vi "Lab Panel V4.90.vi"() -> ()   [LabVIEW 2013] (continued)
              n212 = Bundle(cluster=w241, "Tmp Live"=w237, "Tmp Neut"=w236) -> (w239:T2)  [unwired: 3 in]
              n213 = local write "TEMP LA02"(w243) -> ()
              n214 = local write "SIG LAB02-1"(w239) -> ()
              n215 = local write "SIG LAB02-2"(w238) -> ()
            }
            frame #4 {
              w254 = 0
              n216 = local read "LAB03 TEMP"() -> (w256:T12)
              n217 = Unbundle By Name(w256) -> ("T1 Live"=w249:dbl, "T1 Neut"=w248:dbl, "T2 Live"=w247:dbl, "T2 Neut"=w246:dbl)  [unwired: 2 out]
              n218 = local read "SIG LAB03-1"() -> (w253:T2)
              n219 = local read "SIG LAB03-2"() -> (w252:T2)
              n220 = local read "TEMP LA03"() -> (w257:T9)
              n221 = Bundle By Name(cluster=w257, "TL-1"=w249, "TN-1"=w248, "TL-2"=w247, "TN-2"=w246, "TL -1COUNT"=w254, "TN-1 COUNT"=w254, "TL-2 COUNT"=w254, "TN-2 COUNT"=w254) -> (w255:T9)
              n222 = Bundle(cluster=w252, "Tmp Live"=w247, "Tmp Neut"=w246) -> (w250:T2)  [unwired: 3 in]
              n223 = Bundle(cluster=w253, "Tmp Live"=w249, "Tmp Neut"=w248) -> (w251:T2)  [unwired: 3 in]
              n224 = local write "TEMP LA03"(w255) -> ()
              n225 = local write "SIG LAB03-2"(w250) -> ()
              n226 = local write "SIG LAB03-1"(w251) -> ()
            }
            frame #5 {
              w266 = 0
              n227 = local read "LAB04 TEMP"() -> (w268:T12)
              n228 = Unbundle By Name(w268) -> ("T1 Live"=w261:dbl, "T1 Neut"=w260:dbl, "T2 Live"=w259:dbl, "T2 Neut"=w258:dbl)  [unwired: 2 out]
              n229 = local read "SIG LAB04-2"() -> (w264:T2)
              n230 = local read "SIG LAB04-1"() -> (w265:T2)
              n231 = local read "TEMP LA04"() -> (w269:T9)
              n232 = Bundle By Name(cluster=w269, "TL-1"=w261, "TN-1"=w260, "TL-2"=w259, "TN-2"=w258, "TL -1COUNT"=w266, "TN-1 COUNT"=w266, "TL-2 COUNT"=w266, "TN-2 COUNT"=w266) -> (w267:T9)
              n233 = Bundle(cluster=w264, "Tmp Live"=w259, "Tmp Neut"=w258) -> (w262:T2)  [unwired: 3 in]
              n234 = Bundle(cluster=w265, "Tmp Live"=w261, "Tmp Neut"=w260) -> (w263:T2)  [unwired: 3 in]
              n235 = local write "SIG LAB04-2"(w262) -> ()
              n236 = local write "TEMP LA04"(w267) -> ()
              n237 = local write "SIG LAB04-1"(w263) -> ()
            }
            frame #6 {
              w278 = 0
              n238 = local read "LAB05 TEMP"() -> (w280:T12)
              n239 = Unbundle By Name(w280) -> ("T1 Live"=w273:dbl, "T1 Neut"=w272:dbl, "T2 Live"=w271:dbl, "T2 Neut"=w270:dbl)  [unwired: 2 out]
              n240 = local read "SIG LAB05-2"() -> (w276:T2)
              n241 = local read "SIG LAB05-1"() -> (w277:T2)
              n242 = local read "TEMP LA05"() -> (w281:T9)
              n243 = Bundle By Name(cluster=w281, "TL-1"=w273, "TN-1"=w272, "TL-2"=w271, "TN-2"=w270, "TL -1COUNT"=w278, "TN-1 COUNT"=w278, "TL-2 COUNT"=w278, "TN-2 COUNT"=w278) -> (w279:T9)
              n244 = Bundle(cluster=w276, "Tmp Live"=w271, "Tmp Neut"=w270) -> (w274:T2)  [unwired: 3 in]
              n245 = Bundle(cluster=w277, "Tmp Live"=w273, "Tmp Neut"=w272) -> (w275:T2)  [unwired: 3 in]
              n246 = local write "SIG LAB05-2"(w274) -> ()
              n247 = local write "SIG LAB05-1"(w275) -> ()
              n248 = local write "TEMP LA05"(w279) -> ()
            }
          }
        }
        frame #8 {
          # "enable front panel, all settings done"
          n249 = property on="Tab Control 2" class="TabCtl (strict)"("DisabledEnum"=T16."Enabled" ("Disabled")) -> ()  [unwired: 2 in, 2 out]
          n250 = property on="Tab Control 2" class="TabCtl (strict)"("Value"=0) -> ()  [unwired: 2 in, 2 out]
        }
        frame #9 {
          n251 = property on="Tab Control 2" class="TabCtl (strict)"("Value"=0) -> ()  [unwired: 2 in, 2 out]
        }
      }
    }
    frame #2 {
      n252 = node-c288("loop  delay(mS)") -> (w287:T17)  [unwired: 3 in]
      n253 = timed-loop {
        timing: w287 -> [_]
        timing-out: [_] -> w286
        i -> [w309]
        stop <- "stop" stop-if-true
        n254 = node-c288() -> ()  [unwired: 1 in, 1 out]
        n255 = global write "Global display 1.vi" "stop disp"("stop") -> ()
        n256 = local read "SELECT LAB05-2"() -> (w289:T3)
        n257 = local read "SELECT LAB05-1"() -> (w290:T3)
        n258 = local read "SELECT LAB04-2"() -> (w291:T3)
        n259 = local read "SELECT LAB03-1"() -> (w294:T3)
        n260 = local read "SELECT LAB02-2"() -> (w295:T3)
        n261 = local read "SELECT LAB01-1"() -> (w298:T3)
        n262 = local read "SELECT LAB03-2"() -> (w293:T3)
        n263 = local read "SELECT LAB01-2"() -> (w297:T3)
        n264 = local read "SELECT LAB04-1"() -> (w292:T3)
        n265 = local read "SELECT LAB02-1"() -> (w296:T3)
        n266 = local read "run lab03-2"() -> (w303:bool)
        n267 = local read "run lab04-1"() -> (w302:bool)
        n268 = local read "run lab05-1"() -> (w300:bool)
        n269 = local read "run lab04-2"() -> (w301:bool)
        n270 = local read "run lab05-2"() -> (w299:bool)
        n271 = local read "run lab03-1"() -> (w304:bool)
        n272 = local read "run lab02-2"() -> (w305:bool)
        n273 = local read "run lab02-1"() -> (w306:bool)
        n274 = local read "run lab01-1"() -> (w308:bool)
        n275 = local read "run lab01-2"() -> (w307:bool)
        n276 = stacked-sequence {
          seq-local: [_ w374 _ _ _ _ _ _ _ _ _ _ _ _ _ _ _ _ _ _ _ _ _] -> [_ _ _ _ _ w2475 _ _ _ _ _ _ _ _ _ _ _ _ _ _ _ _ _]
          seq-local: [_ w373 _ _ _ _ _ _ _ _ _ _ _ _ _ _ _ _ _ _ _ _ _] -> [_ _ _ _ _ w2474 _ _ _ _ _ _ _ _ _ _ _ _ _ _ _ _ _]
          seq-local: [_ w360 _ _ _ _ _ _ _ _ _ _ _ _ _ _ _ _ _ _ _ _ _] -> [_ _ _ _ _ w2473 _ _ _ _ _ _ _ _ _ _ _ _ _ _ _ _ _]
          seq-local: [_ w359 _ _ _ _ _ _ _ _ _ _ _ _ _ _ _ _ _ _ _ _ _] -> [_ _ _ _ _ w2472 _ _ _ _ _ _ _ _ _ _ _ _ _ _ _ _ _]
          seq-local: [_ w358 _ _ _ _ _ _ _ _ _ _ _ _ _ _ _ _ _ _ _ _ _] -> [_ _ _ _ _ w2471 _ _ _ _ _ _ _ _ _ _ _ _ _ _ _ _ _]
          seq-local: [_ w357 _ _ _ _ _ _ _ _ _ _ _ _ _ _ _ _ _ _ _ _ _] -> [_ _ _ _ _ w2470 _ _ _ _ _ _ _ _ _ _ _ _ _ _ _ _ _]
          seq-local: [_ w356 _ _ _ _ _ _ _ _ _ _ _ _ _ _ _ _ _ _ _ _ _] -> [_ _ _ _ _ w2469 _ _ _ _ _ _ _ _ _ _ _ _ _ _ _ _ _]
          seq-local: [_ w355 _ _ _ _ _ _ _ _ _ _ _ _ _ _ _ _ _ _ _ _ _] -> [_ _ _ _ _ w2468 _ _ _ _ _ _ _ _ _ _ _ _ _ _ _ _ _]
          seq-local: [_ w354 _ _ _ _ _ _ _ _ _ _ _ _ _ _ _ _ _ _ _ _ _] -> [_ _ _ _ _ w2467 _ _ _ _ _ _ _ _ _ _ _ _ _ _ _ _ _]
          seq-local: [_ w353 _ _ _ _ _ _ _ _ _ _ _ _ _ _ _ _ _ _ _ _ _] -> [_ _ _ _ _ w2466 _ _ _ _ _ _ _ _ _ _ _ _ _ _ _ _ _]
          tunnel: w308 -> [_ _ w390 w638 w2065 w2495 w2810 w3297 _ _ _ _ w3722 _ w4679 _ _ w4966 w5269 w5451 _ _ _]
          tunnel: w307 -> [_ _ w389 w636 w2064 w2494 w2811 w3296 _ _ _ _ w3721 _ w4677 _ _ w4965 w5268 w5449 _ _ _]
          tunnel: w306 -> [_ _ w388 w634 w2063 w2493 w2809 w3295 _ _ _ _ w3720 _ w4675 _ _ w4964 w5267 w5448 _ _ _]
          tunnel: w305 -> [_ _ w387 w632 w2062 w2492 w2808 w3294 _ _ _ _ w3719 _ w4673 _ _ w4963 w5266 w5447 _ _ _]
          tunnel: w304 -> [_ _ w386 w630 w2061 w2491 w2807 w3293 _ _ _ _ w3718 _ w4671 _ _ w4962 w5265 w5446 _ _ _]
          tunnel: w303 -> [_ _ w385 w628 w2060 w2490 w2806 w3292 _ _ _ _ w3717 _ w4669 _ _ w4961 w5264 w5445 _ _ _]
          tunnel: w302 -> [_ _ w384 w626 w2059 w2489 w2805 w3291 _ _ _ _ w3716 _ w4667 _ _ w4960 w5263 w5444 _ _ _]
          tunnel: w301 -> [_ _ w383 w624 w2058 w2488 w2804 w3290 _ _ _ _ w3715 _ w4665 _ _ w4959 w5262 w5443 _ _ _]
          tunnel: w300 -> [_ _ w382 w622 w2057 w2487 w2803 w3289 _ _ _ _ w3714 _ w4663 _ _ w4958 w5261 w5442 _ _ _]
          tunnel: w299 -> [_ _ w381 w620 w2056 w2486 w2802 w3288 _ _ _ _ w3713 _ w4661 _ _ w4957 w5260 w5441 _ _ _]
          tunnel: w298 -> [_ _ _ w637 w2055 w2485 _ _ _ _ _ _ _ _ w4681 _ _ _ _ _ w5789 _ _]
          tunnel: w297 -> [_ _ _ w635 w2054 w2484 _ _ _ _ _ _ _ _ w4676 _ _ _ _ _ w5788 _ _]
          tunnel: w296 -> [_ _ _ w633 w2053 w2483 _ _ _ _ _ _ _ _ w4674 _ _ _ _ _ w5787 _ _]
          tunnel: w295 -> [_ _ _ w631 w2052 w2482 _ _ _ _ _ _ _ _ w4672 _ _ _ _ _ w5786 _ _]
          tunnel: w294 -> [_ _ _ w629 w2051 w2481 _ _ _ _ _ _ _ _ w4670 _ _ _ _ _ w5785 _ _]
          tunnel: w293 -> [_ _ _ w627 w2050 w2480 _ _ _ _ _ _ _ _ w4668 _ _ _ _ _ w5784 _ _]
          tunnel: w292 -> [_ _ _ w625 w2049 w2479 _ _ _ _ _ _ _ _ w4666 _ _ _ _ _ w5783 _ _]
          tunnel: w291 -> [_ _ _ w623 w2048 w2478 _ _ _ _ _ _ _ _ w4664 _ _ _ _ _ w5782 _ _]
          tunnel: w290 -> [_ _ _ w621 w2047 w2477 _ _ _ _ _ _ _ _ w4662 _ _ _ _ _ w5781 _ _]
          tunnel: w289 -> [_ _ _ w619 w2046 w2476 _ _ _ _ _ _ _ _ w4660 _ _ _ _ _ w5780 _ _]
          frame #0 {
            w316 = FALSE
            w321 = 0.5
            # "set up cycle control"
            n277 = local read "jig cycle"() -> (w320:dbl)
            n278 = local read "Amps Fail level"() -> (w314:dbl)
            n279 = Divide(x="JIG ON TIME (S)", y=w321) -> (x/y=→"on loops":dbl)
            n280 = Divide(x="JIG OFF TIME (S)", y=w321) -> (x/y=→"off loops":dbl)
            n281 = global write "Global display 3.vi" "Amps Fail"(w314) -> ()
            n282 = Increment(x=w320) -> (x+1=w319:dbl)
            n283 = local write "TEMP"(w316) -> ()
            n284 = local write "AI"(w316) -> ()
            n285 = local read "Network Directory"() -> (w313:path)
            n286 = local write "jig cycle"(w319) -> ()
            n287 = call "sub vi - check network dir v2.vi"("PATH"=w313) -> ("error"=w312:bool)  [unwired: 10 in]
            n288 = local write "network error"(w312) -> ()
            n289 = global write "Global display 3.vi" "network drive"(w312) -> ()
            n290 = event shown="[1] \"ADMIN\": Value Change" {
              selector: _ -> [_ _]
              dyn-events: _ -> [_ _]
              timeout: 10 -> [_ _]
              event Timeout {
                n291 = event-data() -> ()  [unwired: 1 in, 3 out]
              }
              event "ADMIN": Value Change {
                n292 = event-data() -> ()  [unwired: 1 in, 6 out]
                n293 = stacked-sequence {
                  seq-local: [_ w325 _] -> [_ _ w326]
                  frame #0 {
                    n294 = global write "Global 1.vi" "password"("9949") -> ()
                  }
                  frame #1 {
                    n295 = call "sub vi - password 1.vi"() -> ("RESULT"=w325:bool)  [unwired: 11 in]
                  }
                  frame #2 {
                    w328 = FALSE
                    n296 = property on="Tab Control 2" class="TabCtl (strict)"() -> ("Pages"=w332:refnum<vi>[])  [unwired: 2 in, 2 out]
                    n297 = Select(t=TRUE, s=w326, f=w328) -> (s? t:f=w327:bool)
                    n298 = Index Array(array=w332, index=8) -> (element=w330:refnum<vi>)
                    n299 = property class="Page"(reference=w330, "PageVis"=w327) -> ()  [unwired: 1 in, 2 out]
                    n300 = local write "ADMIN"(w328) -> ()
                  }
                }
              }
            }
          }
          frame #1 {
            w370 = 60.0
            # "convert temperature rise minutes to cycles"
            n301 = local read "SET LAB05-2"() -> (w334:T5)
            n302 = local read "SET LAB05-1"() -> (w336:T5)
            n303 = local read "SET LAB04-2"() -> (w338:T5)
            n304 = local read "SET LAB01-1"() -> (w352:T5)
            n305 = local read "SET LAB01-2"() -> (w350:T5)
            n306 = local read "SET LAB02-2"() -> (w346:T5)
            n307 = local read "SET LAB04-1"() -> (w340:T5)
            n308 = local read "SET LAB03-1"() -> (w344:T5)
            n309 = local read "SET LAB03-2"() -> (w342:T5)
            n310 = local read "SET LAB02-1"() -> (w348:T5)
            n311 = local read "JIG OFF TIME (S)"() -> (w375:dbl)
            n312 = local read "JIG ON TIME (S)"() -> (w376:dbl)
            n313 = Unbundle(w334) -> ("T-RISE mins"=w333:dbl)  [unwired: 4 out]
            n314 = Unbundle(w336) -> ("T-RISE mins"=w335:dbl)  [unwired: 4 out]
            n315 = Unbundle(w352) -> ("T-RISE mins"=w351:dbl)  [unwired: 4 out]
            n316 = Unbundle(w338) -> ("T-RISE mins"=w337:dbl)  [unwired: 4 out]
            n317 = Unbundle(w350) -> ("T-RISE mins"=w349:dbl)  [unwired: 4 out]
            n318 = Unbundle(w348) -> ("T-RISE mins"=w347:dbl)  [unwired: 4 out]
            n319 = Unbundle(w340) -> ("T-RISE mins"=w339:dbl)  [unwired: 4 out]
            n320 = Unbundle(w346) -> ("T-RISE mins"=w345:dbl)  [unwired: 4 out]
            n321 = Unbundle(w342) -> ("T-RISE mins"=w341:dbl)  [unwired: 4 out]
            n322 = Unbundle(w344) -> ("T-RISE mins"=w343:dbl)  [unwired: 4 out]
            n323 = Add(x=w376, y=w375) -> (x+y=w369:dbl)
            n324 = Multiply(x=w370, y=w341) -> (x*y=w365:dbl)
            n325 = Multiply(x=w370, y=w339) -> (x*y=w364:dbl)
            n326 = Multiply(x=w370, y=w337) -> (x*y=w363:dbl)
            n327 = Multiply(x=w370, y=w335) -> (x*y=w362:dbl)
            n328 = Multiply(x=w370, y=w333) -> (x*y=w361:dbl)
            n329 = Multiply(x=w370, y=w349) -> (x*y=w371:dbl)
            n330 = Multiply(x=w370, y=w343) -> (x*y=w366:dbl)
            n331 = Multiply(x=w370, y=w351) -> (x*y=w372:dbl)
            n332 = Multiply(x=w370, y=w347) -> (x*y=w368:dbl)
            n333 = Multiply(x=w370, y=w345) -> (x*y=w367:dbl)
            n334 = Divide(x=w362, y=w369) -> (x/y=w354:dbl)
            n335 = Divide(x=w363, y=w369) -> (x/y=w355:dbl)
            n336 = Divide(x=w364, y=w369) -> (x/y=w356:dbl)
            n337 = Divide(x=w361, y=w369) -> (x/y=w353:dbl)
            n338 = Divide(x=w366, y=w369) -> (x/y=w358:dbl)
            n339 = Divide(x=w372, y=w369) -> (x/y=w374:dbl)
            n340 = Divide(x=w371, y=w369) -> (x/y=w373:dbl)
            n341 = Divide(x=w368, y=w369) -> (x/y=w360:dbl)
            n342 = Divide(x=w367, y=w369) -> (x/y=w359:dbl)
            n343 = Divide(x=w365, y=w369) -> (x/y=w357:dbl)
          }
          frame #2 {
            # "control cycle loops"
            n344 = local read "JIG OFF TIME (S)"() -> (w379:dbl)
            n345 = local read "JIG ON TIME (S)"() -> (w378:dbl)
            n346 = local read "jig cycle"() -> (w392:dbl)
            n347 = local read "on loops"() -> (w394:dbl)
            n348 = local read "off loops"() -> (w393:dbl)
            n349 = Add(x=w379, y=w378) -> (x+y=w377:dbl)
            n350 = Add(x=w394, y=w393) -> (x+y=w380:dbl)
            n351 = Greater Or Equal?(x=w392, y=w380) -> (x >= y?=w391:bool)
            n352 = case shown="True" w391 {
              tunnel: w390 -> [_ w428]
              tunnel: w389 -> [_ w427]
              tunnel: w388 -> [_ w426]
              tunnel: w387 -> [_ w425]
              tunnel: w386 -> [_ w424]
              tunnel: w385 -> [_ w423]
              tunnel: w384 -> [_ w422]
              tunnel: w383 -> [_ w421]
              tunnel: w382 -> [_ w420]
              tunnel: w381 -> [_ w419]
              tunnel: w377 -> [_ w418]
              frame False {
              }
              frame True {
                # "increment cycle value and convert cycles to minutes for temp rise"
                n353 = stacked-sequence {
                  frame #0 {
                    n354 = local read "Panel #"() -> (w431:dbl)
                    n355 = Increment(x=w431) -> (x+1=w430:dbl)
                    n356 = local write "Panel #"(w430) -> ()
                  }
                  frame #1 {
                    n357 = local read "Panel #"() -> (w432:dbl)
                    n358 = Greater?(x=w432, y=5) -> (0:w434:bool)
                    n359 = case shown="True" w434 {
                      frame False {
                      }
                      frame True {
                        n360 = local write "Panel #"(1) -> ()
                      }
                    }
                  }
                }
                n361 = local read "JIG RELAY CYCLES"() -> (w417:T8)
                n362 = local read "Panel #"() -> (→"Tmp Upd":dbl)
                n363 = Unbundle By Name(w417) -> ("LAB01-1"=w415:dbl, "LAB01-2"=w413:dbl, "LAB02-1"=w411:dbl, "LAB02-2"=w409:dbl, "LAB03-1"=w407:dbl, "LAB03-2"=w405:dbl, "LAB04-1"=w403:dbl, "LAB04-2"=w401:dbl, "LAB05-1"=w399:dbl, "LAB05-2"=w397:dbl)
                n364 = stacked-sequence {
                  tunnel: w428 -> [w446 _ _ _ _ _ _ _ _ _]
                  tunnel: w427 -> [_ w463 _ _ _ _ _ _ _ _]
                  tunnel: w426 -> [_ _ w480 _ _ _ _ _ _ _]
                  tunnel: w425 -> [_ _ _ w497 _ _ _ _ _ _]
                  tunnel: w424 -> [_ _ _ _ w514 _ _ _ _ _]
                  tunnel: w423 -> [_ _ _ _ _ w531 _ _ _ _]
                  tunnel: w422 -> [_ _ _ _ _ _ w548 _ _ _]
                  tunnel: w421 -> [_ _ _ _ _ _ _ w565 _ _]
                  tunnel: w420 -> [_ _ _ _ _ _ _ _ w582 _]
                  tunnel: w419 -> [_ _ _ _ _ _ _ _ _ w599]
                  tunnel: w418 -> [w443 w460 w477 w494 w511 w528 w545 w562 w579 w596]
                  tunnel: w415 -> [w437 _ _ _ _ _ _ _ _ _]
                  tunnel: [w436 _ _ _ _ _ _ _ _ _] -> w414
                  tunnel: w413 -> [_ w454 _ _ _ _ _ _ _ _]
                  tunnel: [_ w453 _ _ _ _ _ _ _ _] -> w412
                  tunnel: w411 -> [_ _ w471 _ _ _ _ _ _ _]
                  tunnel: [_ _ w470 _ _ _ _ _ _ _] -> w410
                  tunnel: w409 -> [_ _ _ w488 _ _ _ _ _ _]
                  tunnel: [_ _ _ w487 _ _ _ _ _ _] -> w408
                  tunnel: w407 -> [_ _ _ _ w505 _ _ _ _ _]
                  tunnel: [_ _ _ _ w504 _ _ _ _ _] -> w406
                  tunnel: w405 -> [_ _ _ _ _ w522 _ _ _ _]
                  tunnel: [_ _ _ _ _ w521 _ _ _ _] -> w404
                  tunnel: w403 -> [_ _ _ _ _ _ w539 _ _ _]
                  tunnel: [_ _ _ _ _ _ w538 _ _ _] -> w402
                  tunnel: w401 -> [_ _ _ _ _ _ _ w556 _ _]
                  tunnel: [_ _ _ _ _ _ _ w555 _ _] -> w400
                  tunnel: w399 -> [_ _ _ _ _ _ _ _ w573 _]
                  tunnel: [_ _ _ _ _ _ _ _ w572 _] -> w398
                  tunnel: w397 -> [_ _ _ _ _ _ _ _ _ w590]
                  tunnel: [_ _ _ _ _ _ _ _ _ w589] -> w396
                  frame #0 {
                    n365 = local read "DISP LAB01-1"() -> (w441:T4)
                    n366 = Unbundle(w441) -> ("CYCLE"=w442:dbl)  [unwired: 2 out]
                    n367 = case shown="True" w446 {
                      tunnel: w442 -> [w448 w452]
                      tunnel: [w448 w451] -> w440
                      tunnel: w437 -> [w447 w450]
                      tunnel: [w447 w449] -> w436
                      frame False {
                      }
                      frame True {
                        n368 = Increment(x=w450) -> (x+1=w449:dbl)
                        n369 = Increment(x=w452) -> (x+1=w451:dbl)
                      }
                    }
                    n370 = Multiply(x=w440, y=w443) -> (x*y=w444:dbl)
                    n371 = Divide(x=w444, y=60.0) -> (x/y=w439:dbl)
                    n372 = Bundle(cluster=w441, "CYCLE"=w440, "MINS"=w439) -> (w438:T4)  [unwired: 1 in]
                    n373 = local write "DISP LAB01-1"(w438) -> ()
                  }
                  frame #1 {
                    n374 = local read "DISP LAB01-2"() -> (w458:T4)
                    n375 = Unbundle(w458) -> ("CYCLE"=w459:dbl)  [unwired: 2 out]
                    n376 = case shown="True" w463 {
                      tunnel: w459 -> [w465 w469]
                      tunnel: [w465 w468] -> w456
                      tunnel: w454 -> [w464 w467]
                      tunnel: [w464 w466] -> w453
                      frame False {
                      }
                      frame True {
                        n377 = Increment(x=w467) -> (x+1=w466:dbl)
                        n378 = Increment(x=w469) -> (x+1=w468:dbl)
                      }
                    }
                    n379 = Multiply(x=w456, y=w460) -> (x*y=w461:dbl)
                    n380 = Divide(x=w461, y=60.0) -> (x/y=w455:dbl)
                    n381 = Bundle(cluster=w458, "CYCLE"=w456, "MINS"=w455) -> (w457:T4)  [unwired: 1 in]
                    n382 = local write "DISP LAB01-2"(w457) -> ()
                  }
                  frame #2 {
                    n383 = local read "DISP LAB02-1"() -> (w475:T4)
                    n384 = Unbundle(w475) -> ("CYCLE"=w476:dbl)  [unwired: 2 out]
                    n385 = case shown="True" w480 {
                      tunnel: [w482 w486] -> w473
                      tunnel: w476 -> [w482 w485]
                      tunnel: w471 -> [w481 w484]
                      tunnel: [w481 w483] -> w470
                      frame False {
                      }
                      frame True {
                        n386 = Increment(x=w484) -> (x+1=w483:dbl)
                        n387 = Increment(x=w485) -> (x+1=w486:dbl)
                      }
                    }
                    n388 = Multiply(x=w473, y=w477) -> (x*y=w478:dbl)
                    n389 = Divide(x=w478, y=60.0) -> (x/y=w472:dbl)
                    n390 = Bundle(cluster=w475, "CYCLE"=w473, "MINS"=w472) -> (w474:T4)  [unwired: 1 in]
                    n391 = local write "DISP LAB02-1"(w474) -> ()
                  }
                  frame #3 {
                    n392 = local read "DISP LAB02-2"() -> (w492:T4)
                    n393 = Unbundle(w492) -> ("CYCLE"=w493:dbl)  [unwired: 2 out]
                    n394 = case shown="True" w497 {
                      tunnel: [w499 w503] -> w491
                      tunnel: w493 -> [w499 w502]
                      tunnel: w488 -> [w498 w501]
                      tunnel: [w498 w500] -> w487
                      frame False {
                      }
                      frame True {
                        n395 = Increment(x=w501) -> (x+1=w500:dbl)
                        n396 = Increment(x=w502) -> (x+1=w503:dbl)
                      }
                    }
                    n397 = Multiply(x=w491, y=w494) -> (x*y=w495:dbl)
                    n398 = Divide(x=w495, y=60.0) -> (x/y=w490:dbl)
                    n399 = Bundle(cluster=w492, "CYCLE"=w491, "MINS"=w490) -> (w489:T4)  [unwired: 1 in]
                    n400 = local write "DISP LAB02-2"(w489) -> ()
                  }
                  frame #4 {
                    n401 = local read "DISP LAB03-1"() -> (w509:T4)
                    n402 = Unbundle(w509) -> ("CYCLE"=w510:dbl)  [unwired: 2 out]
                    n403 = case shown="True" w514 {
                      tunnel: [w516 w520] -> w506
                      tunnel: w510 -> [w516 w519]
                      tunnel: w505 -> [w515 w518]
                      tunnel: [w515 w517] -> w504
                      frame False {
                      }
                      frame True {
                        n404 = Increment(x=w518) -> (x+1=w517:dbl)
                        n405 = Increment(x=w519) -> (x+1=w520:dbl)
                      }
                    }
                    n406 = Multiply(x=w506, y=w511) -> (x*y=w512:dbl)
                    n407 = Divide(x=w512, y=60.0) -> (x/y=w507:dbl)
                    n408 = Bundle(cluster=w509, "CYCLE"=w506, "MINS"=w507) -> (w508:T4)  [unwired: 1 in]
                    n409 = local write "DISP LAB03-1"(w508) -> ()
                  }
                  frame #5 {
                    n410 = local read "DISP LAB03-2"() -> (w526:T4)
                    n411 = Unbundle(w526) -> ("CYCLE"=w527:dbl)  [unwired: 2 out]
                    n412 = case shown="True" w531 {
                      tunnel: [w533 w537] -> w525
                      tunnel: w527 -> [w533 w536]
                      tunnel: w522 -> [w532 w535]
                      tunnel: [w532 w534] -> w521
                      frame False {
                      }
                      frame True {
                        n413 = Increment(x=w535) -> (x+1=w534:dbl)
                        n414 = Increment(x=w536) -> (x+1=w537:dbl)
                      }
                    }
                    n415 = Multiply(x=w525, y=w528) -> (x*y=w529:dbl)
                    n416 = Divide(x=w529, y=60.0) -> (x/y=w524:dbl)
                    n417 = Bundle(cluster=w526, "CYCLE"=w525, "MINS"=w524) -> (w523:T4)  [unwired: 1 in]
                    n418 = local write "DISP LAB03-2"(w523) -> ()
                  }
                  frame #6 {
                    n419 = local read "DISP LAB04-1"() -> (w543:T4)
                    n420 = Unbundle(w543) -> ("CYCLE"=w544:dbl)  [unwired: 2 out]
                    n421 = case shown="True" w548 {
                      tunnel: [w550 w554] -> w541
                      tunnel: w544 -> [w550 w553]
                      tunnel: w539 -> [w549 w552]
                      tunnel: [w549 w551] -> w538
                      frame False {
                      }
                      frame True {
                        n422 = Increment(x=w552) -> (x+1=w551:dbl)
                        n423 = Increment(x=w553) -> (x+1=w554:dbl)
                      }
                    }
                    n424 = Multiply(x=w541, y=w545) -> (x*y=w546:dbl)
                    n425 = Divide(x=w546, y=60.0) -> (x/y=w540:dbl)
                    n426 = Bundle(cluster=w543, "CYCLE"=w541, "MINS"=w540) -> (w542:T4)  [unwired: 1 in]
                    n427 = local write "DISP LAB04-1"(w542) -> ()
                  }
                  frame #7 {
                    n428 = local read "DISP LAB04-2"() -> (w560:T4)
                    n429 = Unbundle(w560) -> ("CYCLE"=w561:dbl)  [unwired: 2 out]
                    n430 = case shown="True" w565 {
                      tunnel: [w567 w571] -> w558
                      tunnel: w561 -> [w567 w570]
                      tunnel: w556 -> [w566 w569]
                      tunnel: [w566 w568] -> w555
                      frame False {
                      }
                      frame True {
                        n431 = Increment(x=w569) -> (x+1=w568:dbl)
                        n432 = Increment(x=w570) -> (x+1=w571:dbl)
                      }
                    }
                    n433 = Multiply(x=w558, y=w562) -> (x*y=w564:dbl)
                    n434 = Divide(x=w564, y=60.0) -> (x/y=w557:dbl)
                    n435 = Bundle(cluster=w560, "CYCLE"=w558, "MINS"=w557) -> (w559:T4)  [unwired: 1 in]
                    n436 = local write "DISP LAB04-2"(w559) -> ()
                  }
                  frame #8 {
                    n437 = local read "DISP LAB05-1"() -> (w577:T4)
                    n438 = Unbundle(w577) -> ("CYCLE"=w578:dbl)  [unwired: 2 out]
                    n439 = case shown="True" w582 {
                      tunnel: [w584 w588] -> w575
                      tunnel: w578 -> [w584 w587]
                      tunnel: w573 -> [w583 w586]
                      tunnel: [w583 w585] -> w572
                      frame False {
                      }
                      frame True {
                        n440 = Increment(x=w586) -> (x+1=w585:dbl)
                        n441 = Increment(x=w587) -> (x+1=w588:dbl)
                      }
                    }
                    n442 = Multiply(x=w575, y=w579) -> (x*y=w580:dbl)
                    n443 = Divide(x=w580, y=60.0) -> (x/y=w574:dbl)
                    n444 = Bundle(cluster=w577, "CYCLE"=w575, "MINS"=w574) -> (w576:T4)  [unwired: 1 in]
                    n445 = local write "DISP LAB05-1"(w576) -> ()
                  }
                  frame #9 {
                    n446 = local read "DISP LAB05-2"() -> (w595:T4)
                    n447 = Unbundle(w595) -> ("CYCLE"=w594:dbl)  [unwired: 2 out]
                    n448 = case shown="True" w599 {
                      tunnel: [w601 w605] -> w593
                      tunnel: w594 -> [w601 w604]
                      tunnel: w590 -> [w600 w603]
                      tunnel: [w600 w602] -> w589
                      frame False {
                      }
                      frame True {
                        n449 = Increment(x=w603) -> (x+1=w602:dbl)
                        n450 = Increment(x=w604) -> (x+1=w605:dbl)
                      }
                    }
                    n451 = Multiply(x=w593, y=w596) -> (x*y=w597:dbl)
                    n452 = Divide(x=w597, y=60.0) -> (x/y=w592:dbl)
                    n453 = Bundle(cluster=w595, "CYCLE"=w593, "MINS"=w592) -> (w591:T4)  [unwired: 1 in]
                    n454 = local write "DISP LAB05-2"(w591) -> ()
                  }
                }
                n455 = local write "jig cycle"(0) -> ()
                n456 = Bundle By Name(cluster=w417, "LAB01-1"=w414, "LAB01-2"=w412, "LAB02-1"=w410, "LAB02-2"=w408, "LAB03-1"=w406, "LAB03-2"=w404, "LAB04-1"=w402, "LAB04-2"=w400, "LAB05-1"=w398, "LAB05-2"=w396) -> (w416:T8)
                n457 = local write "JIG RELAY CYCLES"(w416) -> ()
              }
            }
          }
          frame #3 {
            # "START & STOP test RUN switch change, start test if true and stop test if false"
            n458 = Get Date/Time In Seconds() -> (seconds since 1Jan1904=w617:timestamp)
            n459 = local read "C drive data root dir"() -> (w610:path)
            n460 = Format Date/Time String(time format string (%c)="%b\\%a%d", seconds (now)=w617) -> (date/time string=w641:string)  [unwired: 1 in]
            n461 = Format Date/Time String(time format string (%c)="%H%M", seconds (now)=w617) -> (date/time string=w639:string)  [unwired: 1 in]
            n462 = Format Date/Time String(time format string (%c)="LabPanel%Y", seconds (now)=w617) -> (date/time string=w616:string)  [unwired: 1 in]
            n463 = Path To String(path=w610) -> (string=w613:string)
            n464 = global write "Global 1.vi" "C drive root path"(w610) -> ()
            n465 = local read "Ref deg C"() -> (w606:dbl)
            n466 = Concatenate Strings(w613, "\\") -> (w611:string)
            n467 = event shown="[1] \"RUN LAB01-1\": Value Change" {
              selector: _ -> [_ _ _ _ _ _ _ _ _ _ _]
              dyn-events: _ -> [_ _ _ _ _ _ _ _ _ _ _]
              timeout: 10 -> [_ _ _ _ _ _ _ _ _ _ _]
              tunnel: w611 -> [_ w654 w794 w935 w1075 w1215 w1355 w1495 w1635 w1775 w1916]
              tunnel: w641 -> [_ w653 w793 w934 w1074 w1214 w1354 w1494 w1634 w1774 w1915]
              tunnel: w639 -> [_ w651 w792 w933 w1073 w1213 w1353 w1493 w1633 w1773 w1914]
              tunnel: w637 -> [_ w652 _ _ _ _ _ _ _ _ _]
              tunnel: w638 -> [_ _ _ _ _ _ _ _ _ _ _]
              tunnel: w636 -> [_ _ _ _ _ _ _ _ _ _ _]
              tunnel: w635 -> [_ _ w791 _ _ _ _ _ _ _ _]
              tunnel: w634 -> [_ _ _ _ _ _ _ _ _ _ _]
              tunnel: w633 -> [_ _ _ w932 _ _ _ _ _ _ _]
              tunnel: w632 -> [_ _ _ _ _ _ _ _ _ _ _]
              tunnel: w631 -> [_ _ _ _ w1072 _ _ _ _ _ _]
              tunnel: w630 -> [_ _ _ _ _ _ _ _ _ _ _]
              tunnel: w629 -> [_ _ _ _ _ w1212 _ _ _ _ _]
              tunnel: w628 -> [_ _ _ _ _ _ _ _ _ _ _]
              tunnel: w627 -> [_ _ _ _ _ _ w1352 _ _ _ _]
              tunnel: w626 -> [_ _ _ _ _ _ _ _ _ _ _]
              tunnel: w625 -> [_ _ _ _ _ _ _ w1492 _ _ _]
              tunnel: w624 -> [_ _ _ _ _ _ _ _ _ _ _]
              tunnel: w623 -> [_ _ _ _ _ _ _ _ w1632 _ _]
              tunnel: w622 -> [_ _ _ _ _ _ _ _ _ _ _]
              tunnel: w621 -> [_ _ _ _ _ _ _ _ _ w1772 _]
              tunnel: w620 -> [_ _ _ _ _ _ _ _ _ _ _]
              tunnel: w619 -> [_ _ _ _ _ _ _ _ _ _ w1913]
              tunnel: w616 -> [_ w650 w790 w931 w1071 w1211 w1351 w1491 w1631 w1771 w1912]
              tunnel: [_ w649 w789 w930 w1070 w1210 w1350 w1490 w1630 w1770 w1911] -> w614
              tunnel: "RESET CYCLES TO ZERO?" -> [_ w648 w787 w928 w1068 w1208 w1348 w1488 w1628 w1768 w1909]
              tunnel: "YES" -> [_ w647 w786 w927 w1067 w1207 w1347 w1487 w1627 w1767 w1908]
              tunnel: "NO" -> [_ w646 w785 w926 w1066 w1206 w1346 w1486 w1626 w1766 w1907]
              tunnel: w606 -> [_ w643 w784 w924 w1065 w1205 w1345 w1485 w1625 w1765 w1905]
              event Timeout {
                n468 = event-data() -> ()  [unwired: 1 in, 3 out]
              }
              event "RUN LAB01-1": Value Change {
                n469 = event-data() -> ("NewVal"=w644:bool)  [unwired: 1 in, 5 out]
                n470 = local read "SIG LAB01-1"() -> (w645:T2)
                n471 = local write "run lab01-1"(w644) -> ()
                n472 = case shown="True" w644 {
                  tunnel: w654 -> [_ w692]
                  tunnel: w653 -> [_ w691]
                  tunnel: w652 -> [w656 w690]
                  tunnel: w651 -> [_ w689]
                  tunnel: w650 -> [_ w688]
                  tunnel: [w655 w687] -> w649
                  tunnel: w648 -> [_ w686]
                  tunnel: w647 -> [_ w685]
                  tunnel: w646 -> [_ w684]
                  tunnel: w645 -> [_ w683]
                  tunnel: w643 -> [_ w682]
                  frame False {
                    # "stop test"
                    n473 = stacked-sequence {
                      tunnel: w656 -> [_ w668 _]
                      tunnel: [_ w660 _] -> w655
                      frame #0 {
                        n474 = local read "DISP LAB01-1"() -> (w659:T4)
                        n475 = Bundle(cluster=w659, "STATUS"="STOP") -> (w657:T4)  [unwired: 2 in]
                        n476 = local write "DISP LAB01-1"(w657) -> ()
                      }
                      frame #1 {
                        n477 = local read "DISP LAB01-1"() -> (w667:T4)
                        n478 = Unbundle(w667) -> ("CYCLE"=w665:dbl, "MINS"=w666:dbl)  [unwired: 1 out]
                        n479 = case shown="\"CYCLE TEST\"" w668 {
                          tunnel: w666 -> [_ _ w675]
                          tunnel: w665 -> [w673 w674 _]
                          tunnel: [w673 w674 w675] -> w664
                          frame "CHART TEST", Default {
                          }
                          frame "CYCLE TEST" {
                          }
                          frame "T-RISE TEST" {
                          }
                        }
                        n480 = local read "TDMS LAB01-1"() -> (w672:refnum<k34>)
                        n481 = Build Array("STOPPED") -> (w669:string[])
                        n482 = Build Array(w664) -> (w663:dbl[])
                        n483 = TDMS Write(0:w672, 5:"TEST RESULT", 7:w669, 9:w663) -> (4:w661:refnum<k34>, 15:w662:errorcluster)  [unwired: 2 in, 2 out]
                        n484 = TDMS Close(8:w662, 11:w661) -> (0:w660:errorcluster)  [unwired: 1 out]
                      }
                      frame #2 {
                        n485 = stacked-sequence {
                          tunnel: "LAB01-1" -> [w678 w680]
                          frame #0 {
                            n486 = call "sub vi - defrag tdms v1.vi"("panel id"=w678) -> ("error out"=w677:errorcluster)  [unwired: 10 in]
                            n487 = local write "data file error"(w677) -> ()
                          }
                          frame #1 {
                            n488 = call "Save data file (stop) v3.vi"("panel id"=w680) -> ("network file save error"=w679:errorcluster)  [unwired: 9 in, 1 out]
                            n489 = local write "RESULT LAB01-1"(FALSE) -> ()
                            n490 = local write "data file error"(w679) -> ()
                          }
                        }
                      }
                    }
                  }
                  frame True {
                    n491 = stacked-sequence {
                      seq-local: [w694 _] -> [_ w698]
                      tunnel: w692 -> [_ w708]
                      tunnel: w691 -> [_ w707]
                      tunnel: w690 -> [_ w706]
                      tunnel: w689 -> [_ w705]
                      tunnel: w688 -> [_ w704]
                      tunnel: [_ w703] -> w687
                      tunnel: w686 -> [_ w702]
                      tunnel: w685 -> [_ w701]
                      tunnel: w684 -> [_ w700]
                      tunnel: w683 -> [w696 w699]
                      tunnel: w682 -> [_ w697]
                      frame #0 {
                        n492 = Unbundle(w696) -> ("AMPS"=w695:dbl)  [unwired: 4 out]
                        n493 = call "Check For Amps on v1.vi"("ID"="LAB01-1", "amps"=w695) -> ("amps"=w694:bool)  [unwired: 9 in]
                      }
                      frame #1 {
                        n494 = case shown="True" w698 {
                          tunnel: w708 -> [_ w721]
                          tunnel: w707 -> [_ w720]
                          tunnel: w706 -> [_ w719]
                          tunnel: w705 -> [_ w718]
                          tunnel: w704 -> [_ w717]
                          tunnel: [errorcluster {"status"=FALSE, "code"=0, "source"=""} ("error out") w716] -> w703
                          tunnel: w702 -> [_ w715]
                          tunnel: w701 -> [_ w714]
                          tunnel: w700 -> [_ w713]
                          tunnel: w699 -> [_ w712]
                          tunnel: w697 -> [_ w711]
                          frame False {
                            w709 = FALSE
                            n495 = local write "RUN LAB01-1"(w709) -> ()
                            n496 = local write "run lab01-1"(w709) -> ()
                          }
                          frame True {
                            n497 = stacked-sequence {
                              seq-local: [w722 _ _ _ _] -> [_ w743 _ _ _]
                              tunnel: w721 -> [w727 _ _ _ _]
                              tunnel: w720 -> [w723 _ _ _ _]
                              tunnel: w719 -> [w737 _ _ _ _]
                              tunnel: w718 -> [w730 _ _ _ _]
                              tunnel: w717 -> [w725 _ _ _ _]
                              tunnel: [_ w744 _ _ _] -> w716
                              tunnel: w715 -> [_ _ _ w765 _]
                              tunnel: w714 -> [_ _ _ w775 _]
                              tunnel: w713 -> [_ _ _ w774 _]
                              tunnel: w712 -> [_ _ _ _ _]
                              tunnel: w711 -> [_ _ _ _ w781]
                              frame #0 {
                                w724 = "\\"
                                n498 = case shown="\"CHART TEST\", Default" w737 {
                                tunnel: ["L01-1-CHART TEST-" "L01-1-CYCLE TEST-" "L01-1-T-RISE TEST-"] -> w733
                                frame "CHART TEST", Default {
                                }
                                frame "CYCLE TEST" {
                                }
                                frame "T-RISE TEST" {
                                }
                                }
                                n499 = local read "SET LAB01-1"() -> (w732:T5)
                                n500 = Unbundle(w732) -> ("DESCRIPTION"=w731:string)  [unwired: 4 out]
                                n501 = Concatenate Strings(w727, "\\", w725, w724, w723, w724) -> (w734:string)
                                n502 = String To Path(string=w734) -> (path=w736:path)
                                n503 = Concatenate Strings(w734, w733, w731, "-", w730, ".tdms") -> (w722:string)
                                n504 = Create Folder(path (use dialog)=w736) -> (error out=w735:errorcluster)  [unwired: 2 in, 2 out]
                                n505 = call <vilib>:"Clear Errors.vi"("error in (no error)"=w735) -> ()  [unwired: 6 in, 1 out]
                                n506 = global write "Global 1.vi" "LAB01-1 FILE"(w722) -> ()
                              }
                              frame #1 {
                                (unwired) FALSE
                                n507 = String To Path(string=w743) -> (path=w741:path)
                                n508 = TDMS Open(6:FALSE, 10:T20."create or replace" ("operation (0:open)"), 11:w741) -> (0:w744:errorcluster, 3:→"TDMS LAB01-1":refnum<k34>)  [unwired: 4 in]
                              }
                              frame #2 {
                                n509 = local read "TDMS LAB01-1"() -> (w763:refnum<k34>)
                                n510 = local read "SET LAB01-1"() -> (w752:T5)
                                n511 = Build Array("Testers Name", "Description", "Set Test Cycles", "T-Rise minutes", "T-Rise Deg C") -> (w753:string[])
                                n512 = Unbundle(w752) -> ("NAME"=w751:string, "DESCRIPTION"=w750:string, "CYCLES"=w749:dbl, "T-RISE mins"=w748:dbl, "T-RISE deg C"=w747:dbl)
                                n513 = Number To Decimal String(number=w749) -> (decimal integer string=w762:string)  [unwired: 1 in]
                                n514 = Number To Decimal String(number=w748) -> (decimal integer string=w761:string)  [unwired: 1 in]
                                n515 = Number To Decimal String(number=w747) -> (decimal integer string=w760:string)  [unwired: 1 in]
                                n516 = Build Array(w751, w750, w762, w761, w760) -> (w759:string[])
                                n517 = TDMS Set Properties(5:w759, 7:w753, 11:w763) -> ()  [unwired: 3 in, 4 out]
                              }
                              frame #3 {
                                n518 = local read "DISP LAB01-1"() -> (w773:T4)
                                n519 = Concatenate Strings("LAB01-1  ", w765) -> (w764:string)
                                n520 = Two Button Dialog(message=w764, 1:w774, 2:w775) -> (T button?=w767:bool)
                                n521 = case shown="True" w767 {
                                tunnel: w773 -> [w778 w779]
                                tunnel: [w778 w779] -> w772
                                tunnel: [w777 w780] -> w771
                                tunnel: [w776 w780] -> w770
                                frame False {
                                n522 = Unbundle(w778) -> ("CYCLE"=w777:dbl, "MINS"=w776:dbl)  [unwired: 1 out]
                                }
                                frame True {
                                w780 = 0.0
                                }
                                }
                                n523 = Bundle(cluster=w772, "CYCLE"=w771, "MINS"=w770, "STATUS"="RUN") -> (w769:T4)
                                n524 = local write "DISP LAB01-1"(w769) -> ()
                              }
                              frame #4 {
                                n525 = local read "TEMP START LAB01-1"() -> (w783:cluster{"TL":dbl, "TN":dbl})
                                n526 = Bundle(cluster=w783, "TL"=w781, "TN"=w781) -> (w782:cluster{"TL":dbl, "TN":dbl})
                                n527 = local write "TEMP START LAB01-1"(w782) -> ()
                              }
                            }
                          }
                        }
                      }
                    }
                  }
                }
              }
              event "RUN LAB01-2": Value Change {
                n528 = event-data() -> ("NewVal"=w788:bool)  [unwired: 1 in, 5 out]
                n529 = local write "run lab01-2"(w788) -> ()
                n530 = case shown="True" w788 {
                  tunnel: w794 -> [_ w832]
                  tunnel: w793 -> [_ w831]
                  tunnel: w791 -> [w796 w830]
                  tunnel: w792 -> [_ w829]
                  tunnel: w790 -> [_ w828]
                  tunnel: [w795 w827] -> w789
                  tunnel: w787 -> [_ w826]
                  tunnel: w786 -> [_ w825]
                  tunnel: w785 -> [_ w824]
                  tunnel: w784 -> [_ w822]
                  frame False {
                    # "stop test"
                    n531 = stacked-sequence {
                      tunnel: w796 -> [w805 _]
                      tunnel: [w797 _] -> w795
                      frame #0 {
                        n532 = local read "DISP LAB01-2"() -> (w804:T4)
                        n533 = Unbundle(w804) -> ("CYCLE"=w802:dbl, "MINS"=w803:dbl)  [unwired: 1 out]
                        n534 = case shown="\"CHART TEST\", Default" w805 {
                          tunnel: w803 -> [_ _ w812]
                          tunnel: w802 -> [w810 w811 _]
                          tunnel: [w810 w811 w812] -> w801
                          frame "CHART TEST", Default {
                          }
                          frame "CYCLE TEST" {
                          }
                          frame "T-RISE TEST" {
                          }
                        }
                        n535 = local read "TDMS LAB01-2"() -> (w809:refnum<k34>)
                        n536 = Build Array("STOPPED") -> (w806:string[])
                        n537 = Build Array(w801) -> (w800:dbl[])
                        n538 = TDMS Write(0:w809, 5:"TEST RESULT", 7:w806, 9:w800) -> (4:w798:refnum<k34>, 15:w799:errorcluster)  [unwired: 2 in, 2 out]
                        n539 = TDMS Close(8:w799, 11:w798) -> (0:w797:errorcluster)  [unwired: 1 out]
                      }
                      frame #1 {
                        n540 = local read "DISP LAB01-2"() -> (w816:T4)
                        n541 = stacked-sequence {
                          tunnel: "LAB01-2" -> [w818 w820]
                          frame #0 {
                            n542 = call "sub vi - defrag tdms v1.vi"("panel id"=w818) -> ("error out"=w817:errorcluster)  [unwired: 10 in]
                            n543 = local write "data file error"(w817) -> ()
                          }
                          frame #1 {
                            n544 = call "Save data file (stop) v3.vi"("panel id"=w820) -> ("network file save error"=w819:errorcluster)  [unwired: 9 in, 1 out]
                            n545 = local write "RESULT LAB01-2"(FALSE) -> ()
                            n546 = local write "data file error"(w819) -> ()
                          }
                        }
                        n547 = Bundle(cluster=w816, "STATUS"="STOP") -> (w814:T4)  [unwired: 2 in]
                        n548 = local write "DISP LAB01-2"(w814) -> ()
                      }
                    }
                  }
                  frame True {
                    n549 = local read "SIG LAB01-2"() -> (w823:T2)
                    n550 = stacked-sequence {
                      seq-local: [w834 _] -> [_ w838]
                      tunnel: w832 -> [_ w848]
                      tunnel: w831 -> [_ w847]
                      tunnel: w830 -> [_ w846]
                      tunnel: w829 -> [_ w845]
                      tunnel: w828 -> [_ w844]
                      tunnel: [_ w843] -> w827
                      tunnel: w826 -> [_ w842]
                      tunnel: w825 -> [_ w841]
                      tunnel: w824 -> [_ w840]
                      tunnel: w823 -> [w833 w839]
                      tunnel: w822 -> [_ w837]
                      frame #0 {
                        n551 = Unbundle(w833) -> ("AMPS"=w836:dbl)  [unwired: 4 out]
                        n552 = call "Check For Amps on v1.vi"("ID"="LAB01-2", "amps"=w836) -> ("amps"=w834:bool)  [unwired: 9 in]
                      }
                      frame #1 {
                        n553 = case shown="True" w838 {
                          tunnel: w848 -> [_ w861]
                          tunnel: w847 -> [_ w860]
                          tunnel: w846 -> [_ w859]
                          tunnel: w845 -> [_ w858]
                          tunnel: w844 -> [_ w857]
                          tunnel: [errorcluster {"status"=FALSE, "code"=0, "source"=""} ("error out") w856] -> w843
                          tunnel: w842 -> [_ w855]
                          tunnel: w841 -> [_ w854]
                          tunnel: w840 -> [_ w853]
                          tunnel: w839 -> [_ w852]
                          tunnel: w837 -> [_ w851]
                          frame False {
                            w849 = FALSE
                            n554 = local write "RUN LAB01-2"(w849) -> ()
                            n555 = local write "run lab01-2"(w849) -> ()
                          }
                          frame True {
                            n556 = stacked-sequence {
                              seq-local: [w862 _ _ _ _] -> [_ w886 _ _ _]
                              tunnel: w861 -> [w867 _ _ _ _]
                              tunnel: w860 -> [w864 _ _ _ _]
                              tunnel: w859 -> [w877 _ _ _ _]
                              tunnel: w858 -> [w870 _ _ _ _]
                              tunnel: w857 -> [w865 _ _ _ _]
                              tunnel: [_ w881 _ _ _] -> w856
                              tunnel: w855 -> [_ _ _ w908 _]
                              tunnel: w854 -> [_ _ _ w907 _]
                              tunnel: w853 -> [_ _ _ w906 _]
                              tunnel: w852 -> [_ _ _ _ _]
                              tunnel: w851 -> [_ _ _ _ w921]
                              frame #0 {
                                w863 = "\\"
                                n557 = local read "SET LAB01-2"() -> (w872:T5)
                                n558 = case shown="\"CYCLE TEST\"" w877 {
                                tunnel: ["L01-2-CHART TEST-" "L01-2-CYCLE TEST-" "L01-2-T-RISE TEST-"] -> w873
                                frame "CHART TEST", Default {
                                }
                                frame "CYCLE TEST" {
                                }
                                frame "T-RISE TEST" {
                                }
                                }
                                n559 = Unbundle(w872) -> ("DESCRIPTION"=w871:string)  [unwired: 4 out]
                                n560 = Concatenate Strings(w867, "\\", w865, w863, w864, w863) -> (w874:string)
                                n561 = String To Path(string=w874) -> (path=w876:path)
                                n562 = Concatenate Strings(w874, w873, w871, "-", w870, ".tdms") -> (w862:string)
                                n563 = Create Folder(path (use dialog)=w876) -> (error out=w875:errorcluster)  [unwired: 2 in, 2 out]
                                n564 = call <vilib>:"Clear Errors.vi"("error in (no error)"=w875) -> ()  [unwired: 6 in, 1 out]
                                n565 = global write "Global 1.vi" "LAB01-2 FILE"(w862) -> ()
                              }
                              frame #1 {
                                (unwired) FALSE
                                n566 = String To Path(string=w886) -> (path=w882:path)
                                n567 = TDMS Open(6:FALSE, 10:T20."create or replace" ("operation (0:open)"), 11:w882) -> (0:w881:errorcluster, 3:→"TDMS LAB01-2":refnum<k34>)  [unwired: 4 in]
                              }
                              frame #2 {
                                n568 = local read "SET LAB01-2"() -> (w892:T5)
